vi "Combine.vi"(1 "L":i8 format="%b", 2 "H":i8 format="%b") -> (0 "Out":i16 format="%b")   [LabVIEW 2013]
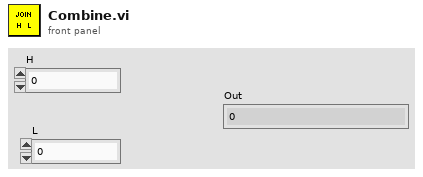
[diagram p1: front panel]
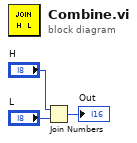
[diagram p0: block diagram]
diagram:
  n1 = Join Numbers(hi="H", lo="L") -> ((hi.lo)=→"Out":u16)
